vi "Write Pref Value.vi"(8 "error in (no error)":errorcluster, 9 "Value":string, 10 "Pref Hierarchy":string[](array[string]), 11 "Pref Group in":refnum<class "Pref Group.lvclass">) -> (0 "error out":errorcluster, 3 "Pref Group out":refnum<class "Pref Group.lvclass">)   [LabVIEW 2020, in "User Prefs.lvlib" / "Pref Group.lvclass"]
uses:
  Pref Group.lvclass
  Pref Group.lvclass/Pref Group.ctl
  lv-cdm/CDM-Config/Config Manager/Config Manager.lvclass
  lv-cdm/CDM-Config/Config Element/Config Element.lvclass
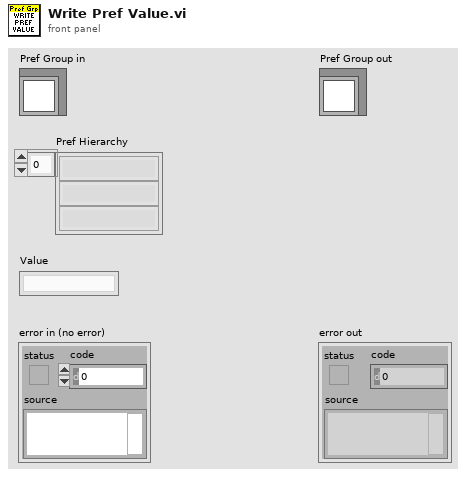
[diagram p1: front panel]
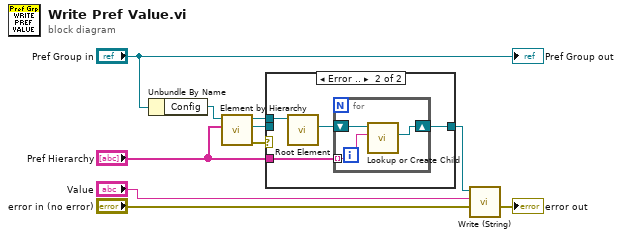
[diagram p0: block diagram]
diagram:
  n1 = Unbundle By Name("Pref Group in") -> ("Config"=w9:refnum<class "Config Manager.lvclass">)
  n2 = call "Element by Hierarchy.vi"("Hierarchy"="Pref Hierarchy", "Config Manager in"=w9) -> ("error out"=w8:errorcluster, "Config Element"=w7:refnum<class "Config Element.lvclass">, "Config Manager out"=w6:refnum<class "Config Manager.lvclass">)  [unwired: 7 in]
  n3 = case shown="Error .." w8 {
    tunnel: w7 -> [w11 _]
    tunnel: [w11 w12] -> w4
    tunnel: w6 -> [_ w15]
    tunnel: "Pref Hierarchy" -> [_ w14]
    frame No Error {
    }
    frame Error {
      n4 = call "Root Element.vi"("Config Manager in"=w15) -> ("Root Element"=w13:refnum<class "Config Element.lvclass">)  [unwired: 8 in, 2 out]
      n5 = for {
        tunnel: w14 -> [w17] mode=indexing
        shift-right: [w16] -> w12
        shift-left: w13 -> [w18]
        n6 = call "Lookup or Create Child.vi"("Name"=w17, "Config Element in"=w18) -> ("Child"=w16:refnum<class "Config Element.lvclass">)  [unwired: 6 in, 3 out]
      }
    }
  }
  n7 = call "Write (String).vi"("error in (no error)"="error in (no error)", "String Value"="Value", "Config Element in"=w4) -> ("error out"=→"error out":errorcluster)  [unwired: 7 in, 1 out]
  "Pref Group out" <- "Pref Group in"
